vi "CameraStartAcquire.vi"(8 "error in (no error)":errorcluster, 11 "NIvision in":refnum<class "IMAQdx.lvclass">) -> (0 "error out":errorcluster, 3 "NIvision out":refnum<class "IMAQdx.lvclass">)   [LabVIEW 2010, in "IMAQdx.lvclass"]
uses:
  IMAQdx.lvclass
  IMAQdx.lvclass/IMAQdx.ctl
  <vilib>/vision/driver/NI_Vision_Acquisition_Software.lvlib
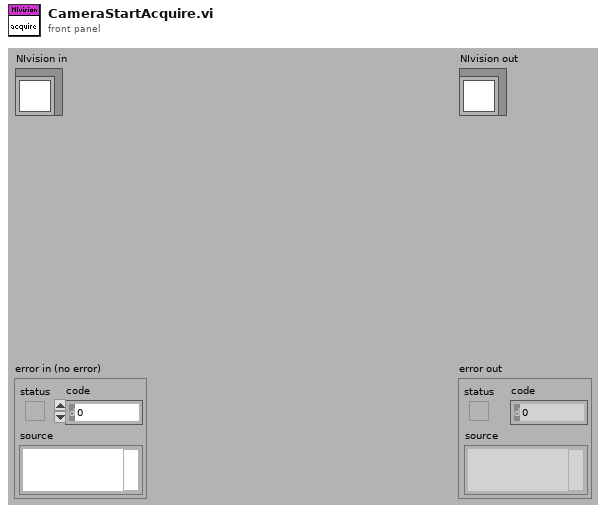
[diagram p1: front panel]
types:
  T1 = typedef "IMAQdx.ctl" = refnum<k21>
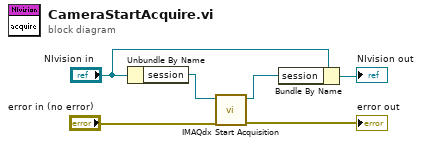
[diagram p0: block diagram]
diagram:
  n1 = Unbundle By Name("NIvision in") -> ("session"=w4:refnum<k21>)
  n2 = call <vilib>:"IMAQdx Start Acquisition.vi"("error in"="error in (no error)", "Session In"=w4) -> ("error out"=→"error out":errorcluster, "Session Out"=w1:T1)  [unwired: 8 in]
  n3 = Bundle By Name(cluster="NIvision in", "session"=w1) -> (→"NIvision out":refnum<class "IMAQdx.lvclass">)
